vi "read_OSC_original_timing.vi"() -> ()   [LabVIEW 2011]
doc: "Demonstrates how to set up an oscilloscope automatically. You can configure this VI to acquire a waveform from a single channel by following the following steps:\n\n1. Specify a valid VISA resource to use. \n2. Specify a channel. \n3. Specify a time-out value for reading a waveform.\n4. Run this VI. The <B>Waveform Graph</B> displays the waveform you acquire."
uses:
  <instrlib>/Tektronix 7000 Series/Tektronix 7000 Series.lvlib
panel:
  out "curve and length command":u32
  out "complete time":u32
  out "meas time (read curve)":u32
  out "fetch waveform timing":u32
  out "overhead":i32
  in  "OSC":refnum<visa-resource-name>="OSC"
  in  "Maximum Time":u32=10000
  out "Waveform Graph":waveform(dbl)(graph)
  in  "STOP":bool
  in  "start":bool
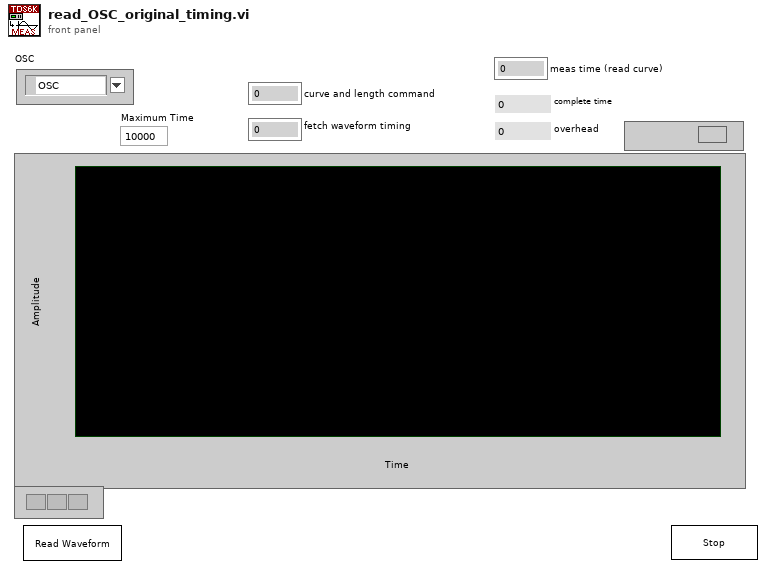
[diagram p1: front panel]
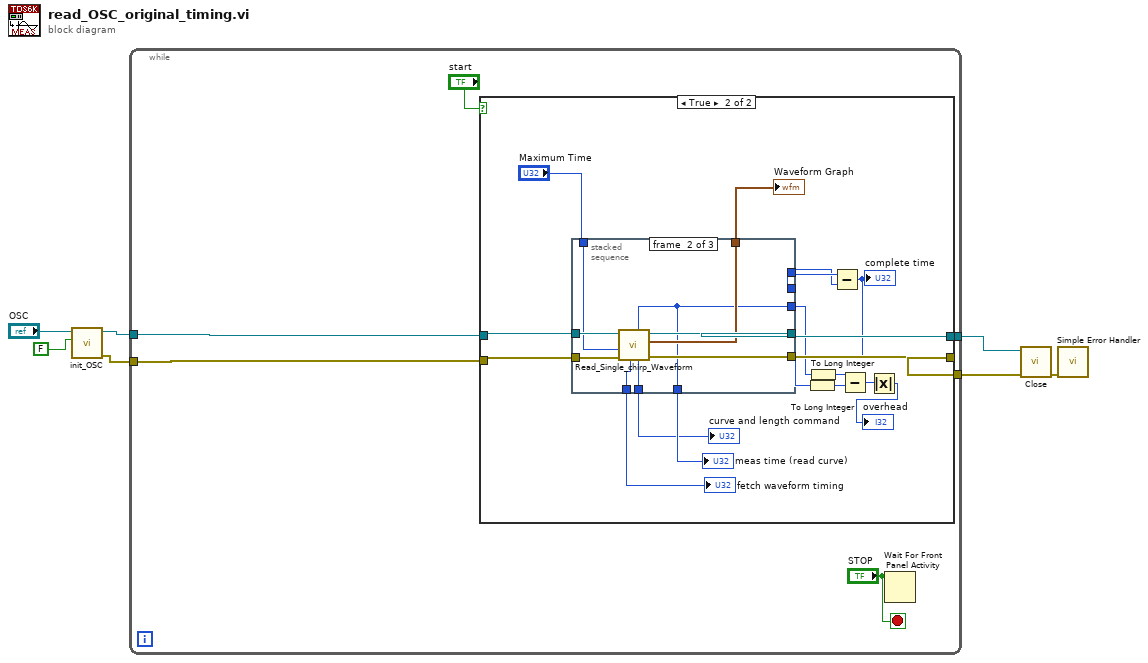
[diagram p0: block diagram]
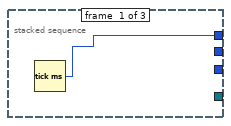
[diagram p3: hidden frame]
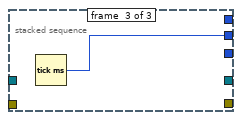
[diagram p4: hidden frame]
diagram:
  n1 = call "init_OSC.vi"("reset (f)"=FALSE, "VISA resource name"="OSC") -> ("error out"=w1:errorcluster, "VISA resource name out"=w2:refnum<visa-resource-name>)  [unwired: 8 in]
  n2 = while {
    tunnel: w2 -> [w9]
    tunnel: w1 -> [w8]
    tunnel: [w11] -> w6
    tunnel: [w10] -> w5
    stop <- "STOP" stop-if-true
    n3 = case shown="True" "start" {
      tunnel: w9 -> [w15 w28]
      tunnel: w8 -> [w14 w29]
      tunnel: [w15 w31] -> w11
      tunnel: [w14 w30] -> w10
      frame False {
      }
      frame True {
        n4 = stacked-sequence {
          tunnel: [_ w42 _] -> w32
          tunnel: [_ w41 _] -> w31
          tunnel: [_ w40 _] -> w30
          tunnel: w29 -> [_ w39 _]
          tunnel: w28 -> [_ w38 _]
          tunnel: "Maximum Time" -> [_ w37 _]
          tunnel: [_ w35 _] -> w23
          tunnel: [_ w36 _] -> w20
          tunnel: [_ w35 _] -> w22
          tunnel: [w33 _ _] -> w18
          tunnel: [_ _ w43] -> w19
          tunnel: [_ w34 _] -> w16
          frame #0 {
            n5 = Tick Count (ms)() -> (millisecond timer value=w33:u32)
          }
          frame #1 {
            n6 = call "Read_Single_chirp_Waveform.vi"("error in (no error)"=w39, "Maximum Time (10000 ms)"=w37, "VISA resource name"=w38) -> ("error out"=w40:errorcluster, "Waveform Data"=w42:waveform(dbl), "VISA resource name out"=w41:refnum<visa-resource-name>, "curve & length command"=w34:u32, "low level meas time"=w35:u32, "fetch waveform timing"=w36:u32)  [unwired: 3 in]
          }
          frame #2 {
            n7 = Tick Count (ms)() -> (millisecond timer value=w43:u32)
          }
        }
        "Waveform Graph" <- w32
        "fetch waveform timing" <- w20
        "meas time (read curve)" <- w22
        "curve and length command" <- w16
        n8 = To Long Integer(number=w23) -> (32bit integer=w26:i32)
        n9 = Subtract(x=w19, y=w18) -> (x-y=w17:u32)
        "complete time" <- w17
        n10 = To Long Integer(number=w17) -> (32bit integer=w25:i32)
        n11 = Subtract(x=w26, y=w25) -> (x-y=w24:i32)
        n12 = Absolute Value(x=w24) -> (abs(x)=→"overhead":i32)
      }
    }
    n13 = Wait For Front Panel Activity(3:"STOP") -> ()  [unwired: 2 in, 1 out]
  }
  n14 = call <instrlib>:"Close.vi"("error in (no error)"=w5, "VISA resource name"=w6) -> ("error out"=w7:errorcluster)  [unwired: 9 in]
  n15 = call <vilib>:"Simple Error Handler.vi"("error in (no error)"=w7) -> ()  [unwired: 4 in, 5 out]
